vi "motionProfileCreatePaths.vi"() -> ()   [LabVIEW 2018]
uses:
  <vilib>/Rock Robotics/WPI/ThirdParty/Phoenix-LabVIEW/Motor Controller/Controls/CTRE_Phoenix_MotorControl_MotionProfileTrajectoryPoint.ctl
  <vilib>/Utility/file.llb/Read Delimited Spreadsheet (DBL).vi
  <vilib>/Rock Robotics/WPI/ThirdParty/Phoenix-LabVIEW/Motor Controller/Closed Loop/Motion Profile/CTRE_Phoenix_MotorControl_BufferedTrajectoryPointStream_WriteAll.vi
  <vilib>/Utility/file.llb/Read Delimited Spreadsheet (string).vi
panel:
  out "Array":T1[](array[typedef])
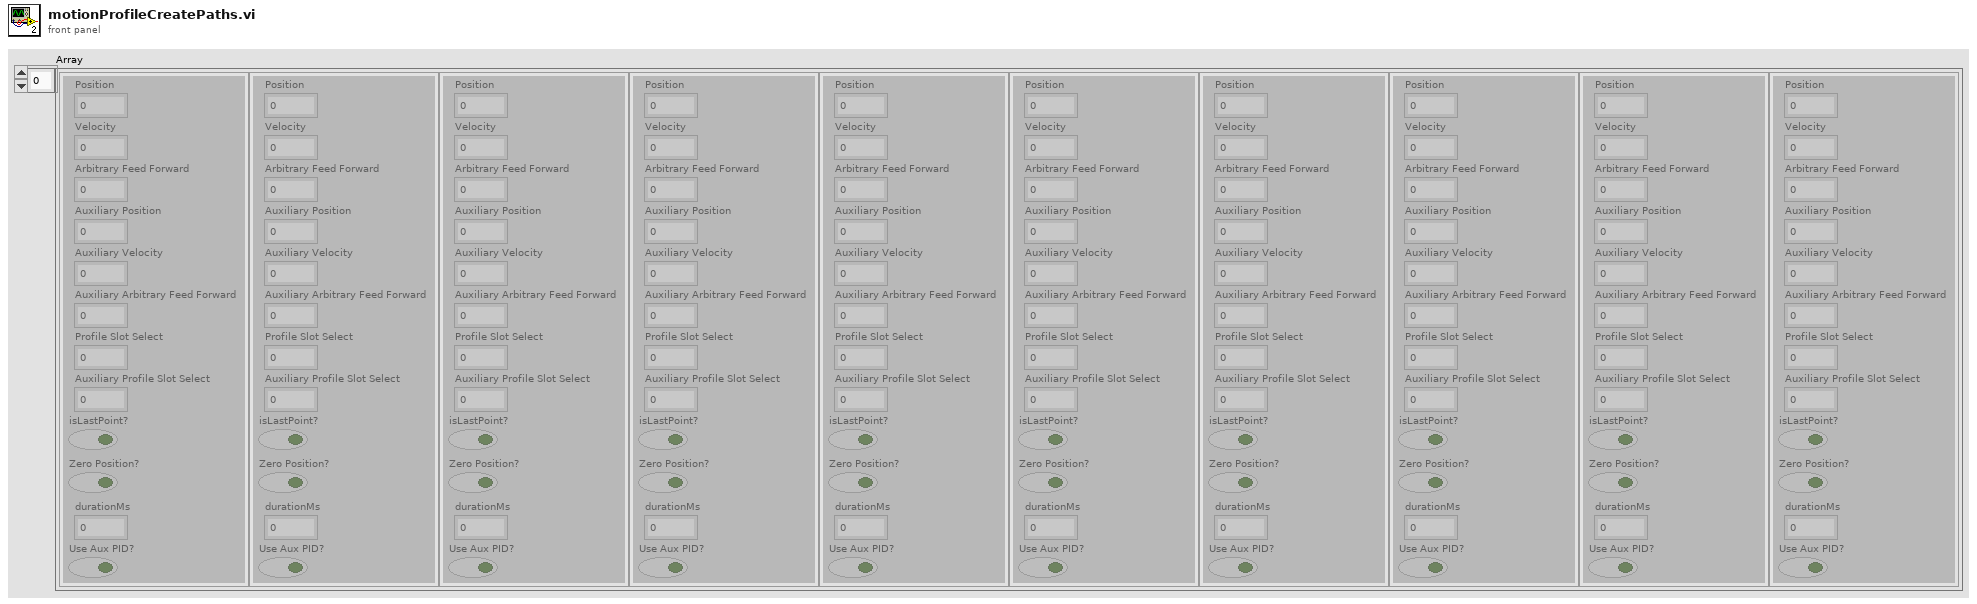
[diagram p1: front panel]
types:
  T1 = typedef "CTRE_Phoenix_MotorControl_MotionProfileTrajectoryPoint.ctl" = cluster{"Position":dbl, "Velocity":dbl, "Arbitrary Feed Forward":dbl, "Auxiliary Position":dbl, "Auxiliary Velocity":dbl, "Auxiliary Arbitrary Feed Forward":dbl, "Profile Slot Select":i32, "Auxiliary Profile Slot Select":i32, "isLastPoint?":bool, "Zero Position?":bool, "durationMs":u32, "Use Aux PID?":bool}
  T2 = enum16{"Inches -> Sensor Units", "Sensor Units -> Inches"}
  T3 = typedef "CTRE_Phoenix_MotorControl_BufferedTrajectoryPointStream_DeviceRef.ctl" = cluster{"Handle":u64, "Library Path":path}
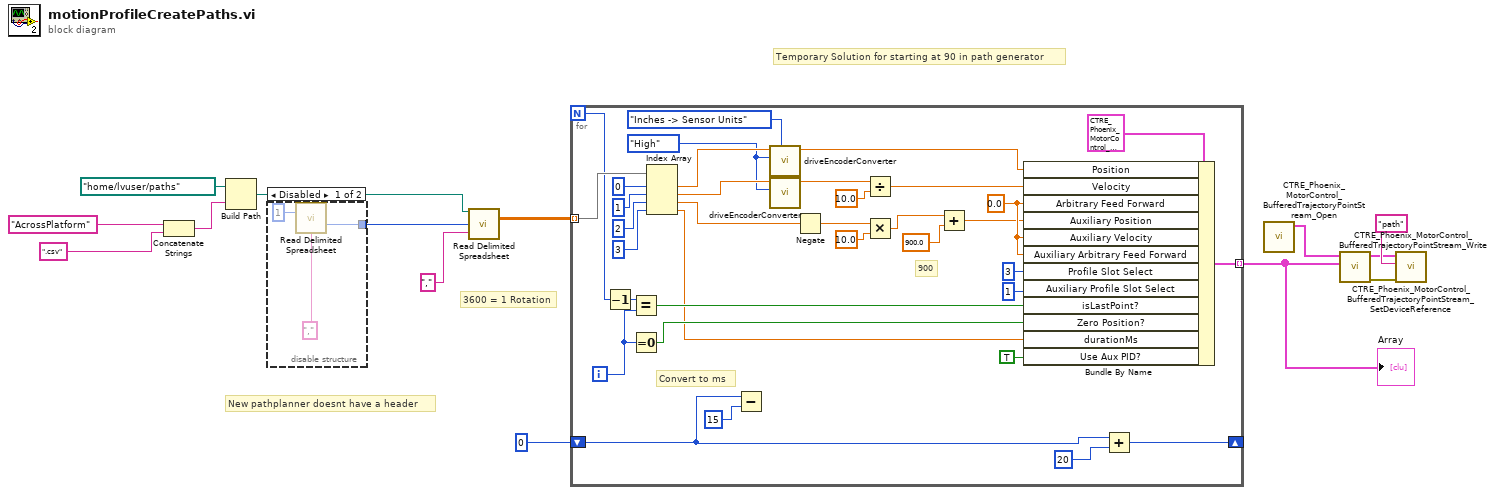
[diagram p0: block diagram]
diagram:
  # "New pathplanner doesnt have a header"
  # "Temporary Solution for starting at 90 in path generator"
  # "3600 = 1 Rotation"
  n1 = Concatenate Strings("AcrossPlatform" ("string"), ".csv") -> (w9:string)
  n2 = Build Path(base path=path "/home/lvuser/paths", name or relative path=w9) -> (appended path=w1:path)
  n3 = disable-structure shown="Disabled" {
    disable-tunnel: [w15 _] -> w8
    frame Disabled {
      n4 = call-poly <vilib>:"Read Delimited Spreadsheet.vi"("number of rows (all:-1)"=1, "delimiter (\\t)"="," ("delimiter (\\t)")) -> ("mark after read (chars.)"=w15:i32)  [unwired: 8 in, 5 out]
    }
    frame Enabled {
    }
  }
  n5 = call-poly <vilib>:"Read Delimited Spreadsheet.vi"("file path (dialog if empty)"=w1, "start of read offset (chars.:0)"=w8, "delimiter (\\t)"="," ("delimiter (\\t)")) -> ("all rows"=w6:dbl[][])  [unwired: 7 in, 5 out]
  n6 = for {
    N -> [w46]
    tunnel: w6 -> [w51] mode=indexing
    tunnel: [w43] -> w3 mode=indexing
    shift-right: [w28] -> _
    shift-left: u32 0 ("durationMs") -> [w26]
    i -> [w40]
    w20 = enum16{"High", "Low"}."High" ("Gear Setting")
    w19 = T2."Inches -> Sensor Units" ("Conversion Direction")
    w50 = 0.0 ("Arbitrary Feed Forward")
    # "900"
    # "Convert to ms"
    n7 = Decrement(x=w46) -> (x-1=w39:i32)
    n8 = Equal?(x=w39, y=w40) -> (x = y?=w47:bool)
    n9 = Equal To 0?(x=w40) -> (x = 0?=w45:bool)
    n10 = Index Array(array=w51, index #1=0 ("index"), index #2=1 ("index"), index #3=2 ("index"), index #4=3 ("index")) -> (element #1=w24:dbl, element #2=w21:dbl, element #3=w34:dbl, element #4=w18:dbl)
    n11 = Subtract(x=w26, y=u32 15) -> ()  [unwired: 1 out]
    n12 = call "driveEncoderConverter.vi"("Conversion Direction"=w19, "Gear Setting"=w20, "Input"=w24) -> ("Output"=w23:dbl)  [unwired: 8 in]
    n13 = call "driveEncoderConverter.vi"("Conversion Direction"=w19, "Gear Setting"=w20, "Input"=w21) -> ("Output"=w22:dbl)  [unwired: 8 in]
    n14 = Negate(x=w34) -> (-x=w29:dbl)
    n15 = Divide(x=w22, y=10.0) -> (x/y=w41:dbl)
    n16 = Multiply(x=w29, y=10.0) -> (x*y=w33:dbl)
    n17 = Add(x=w33, y=900.0) -> (x+y=w31:dbl)
    n18 = Bundle By Name(cluster=T1 {"Position"=0.0, "Velocity"=0.0, "Arbitrary Feed Forward"=0.0, "Auxiliary Position"=0.0, "Auxiliary Velocity"=0.0, "Auxiliary Arbitrary Feed Forward"=0.0, "Profile Slot Select"=0, "Auxiliary Profile Slot Select"=0, "isLastPoint?"=FALSE, "Zero Position?"=FALSE, "durationMs"=0, "Use Aux PID?"=FALSE} ("Trajectory Point"), "Position"=w23, "Velocity"=w41, "Arbitrary Feed Forward"=w50, "Auxiliary Position"=w31, "Auxiliary Velocity"=w50, "Auxiliary Arbitrary Feed Forward"=w50, "Profile Slot Select"=3, "Auxiliary Profile Slot Select"=1, "isLastPoint?"=w47, "Zero Position?"=w45, "durationMs"=w18, "Use Aux PID?"=TRUE) -> (w43:T1)
    n19 = Add(x=w26, y=u32 20) -> (x+y=w28:u32)
  }
  "Array" <- w3
  n20 = call <vilib>:"CTRE_Phoenix_MotorControl_BufferedTrajectoryPointStream_Open.vi"() -> ("BufferedTrajectoryPointStream_DevRef"=w11:T3)  [unwired: 10 in, 1 out]
  n21 = call-poly <vilib>:"CTRE_Phoenix_MotorControl_BufferedTrajectoryPointStream_Write.vi"("Motion Profile Trajectory Point Array"=w3, "BufferedTrajectoryPointStream_DevRef"=w11) -> ("error out"=w13:errorcluster, "BufferedTrajectoryPointStream_DevRef"=w12:T3)  [unwired: 8 in]
  n22 = call <vilib>:"CTRE_Phoenix_MotorControl_BufferedTrajectoryPointStream_SetDeviceReference.vi"("error in (no error)"=w13, "refnum name"="path", "BufferedTrajectoryPointStream_DevRef"=w12) -> ()  [unwired: 7 in, 2 out]
